vi "FTW-TestExecutive-Core_Sequence_Scrub.vi"(0 "FTW-TestExecutive-Core In":refnum<class "FTW-TestExecutive-Core.lvclass">, 11 "error in":errorcluster) -> (4 "FTW-TestExecutive-Core Out":refnum<class "FTW-TestExecutive-Core.lvclass">, 15 "error out":errorcluster)   [LabVIEW 2015, in "FTW-TestExecutive-Core.lvclass"]
uses:
  FTW-TestExecutive-Core.lvclass
  FTW-TestExecutive-Core.lvclass/FTW-TestExecutive-Core.ctl
  FTW-TestExecutive-Step-State.ctl
  FTW-TestExecutive-Results.ctl
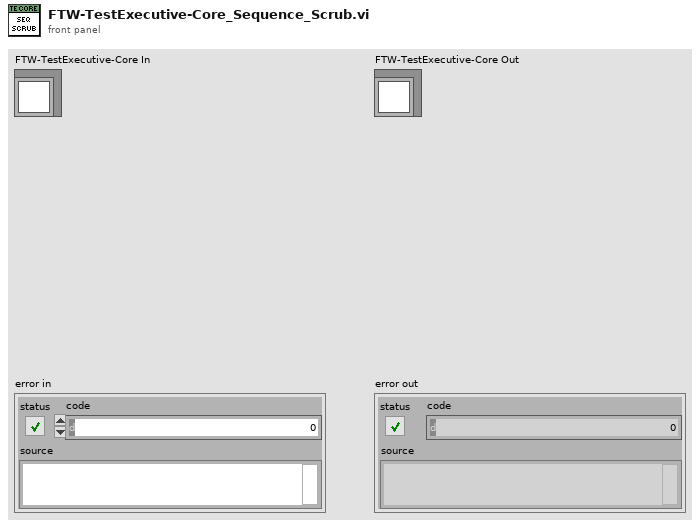
[diagram p1: front panel]
types:
  T1 = typedef "FTW-TestExecutive-Results.ctl" = cluster{"Start Time":timestamp, "Elapsed Time":dbl, "Passed":bool}
  T2 = typedef "FTW-TestExecutive-Step-State.ctl" = enum8{"None", "Failed", "Passed", "Timed out", "Aborted"}
  T3 = typedef "FTW-TestExecutive-Step.ctl" = cluster{"Name":string, "Type":string, "Path":string, "Config":string, "Elapsed Time":dbl, "Passed":bool, "State":T2, "Results":T1}
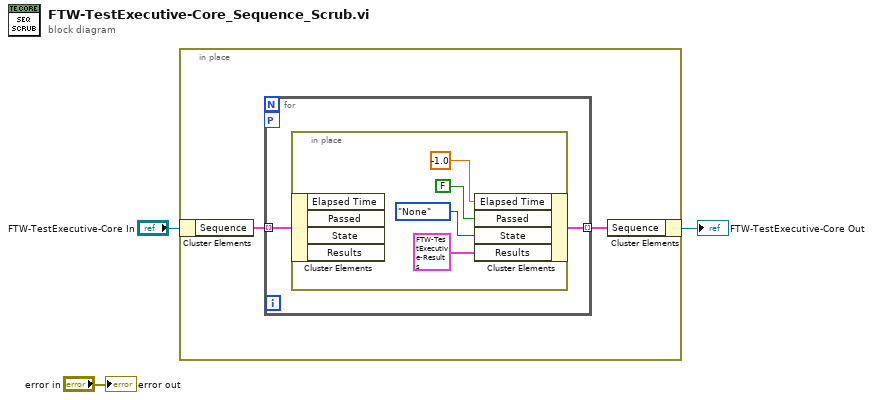
[diagram p0: block diagram]
diagram:
  n1 = in-place {
    n2 = in-place-cluster #1("FTW-TestExecutive-Core In") -> ("Sequence"=w5:T3[])
    n3 = for {
      tunnel: w5 -> [w7] mode=indexing
      workers-P: _ -> [_]
      tunnel: [w6] -> w4 mode=indexing
      n4 = in-place {
        n5 = in-place-cluster #2(w7) -> ()  [unwired: 4 out]
        n6 = in-place-cluster #2("Elapsed Time"=-1.0, "Passed"=FALSE, "State"=FTW-TestExecutive-Step-State."None", "Results"=T1 {"Start Time"=timestamp(0 s since 1904-01-01), "Elapsed Time"=0.0, "Passed"=FALSE}) -> (w6:T3)
      }
    }
    n7 = in-place-cluster #1("Sequence"=w4) -> (→"FTW-TestExecutive-Core Out":refnum<class "FTW-TestExecutive-Core.lvclass">)
  }
  "error out" <- "error in"
